vi "Toggle.vi"(5 "Reinit?":bool, 7 "Initial Value":bool, 11 "In":bool) -> (3 "Toggled":bool)   [LabVIEW 2014]
uses:
  Change Detect Boolean.vi
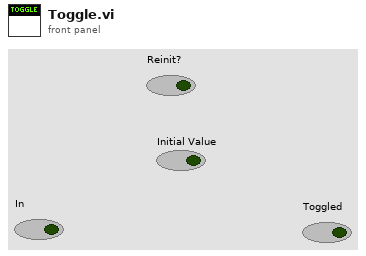
[diagram p1: front panel]
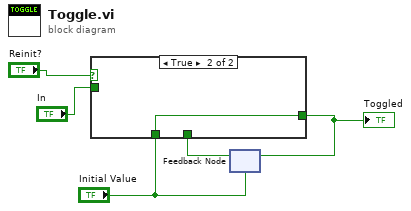
[diagram p0: block diagram]
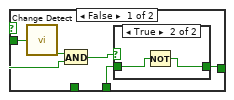
[diagram p2: hidden frame]
diagram:
  n1 = feedback #1("Initial Value") -> (w4:bool)
  n2 = case shown="True" "Reinit?" {
    tunnel: "In" -> [w9 _]
    tunnel: w4 -> [w7 _]
    tunnel: [w6 w14] -> w3
    tunnel: "Initial Value" -> [_ w14]
    frame False {
      n3 = call-poly "Change Detect.vi"("In"=w9) -> ("Changed?"=w10:bool)
      n4 = And(x=w10, y=w9) -> (x .and. y?=w8:bool)
      n5 = case shown="True" w8 {
        tunnel: w7 -> [w11 w12]
        tunnel: [w11 w13] -> w6
        frame False {
        }
        frame True {
          n6 = Not(x=w12) -> (.not. x?=w13:bool)
        }
      }
    }
    frame True {
    }
  }
  "Toggled" <- w3
  n7 = feedback-in #1(w3) -> ()
